vi "LVClass_ComputePhaseSet Read ComputePhaseSet.vi"(8 "error in (no error)":errorcluster, 11 "ComputePhaseSet in":refnum<class "ComputePhaseSet.lvclass">) -> (0 "error out":errorcluster, 2 "ComputePhaseSet":i32, 3 "ComputePhaseSet out":refnum<class "ComputePhaseSet.lvclass">)   [LabVIEW 2020, in "ComputePhaseSet.lvclass"]
uses:
  ComputePhaseSet.lvclass
  ComputePhaseSet.lvclass/ComputePhaseSet.ctl
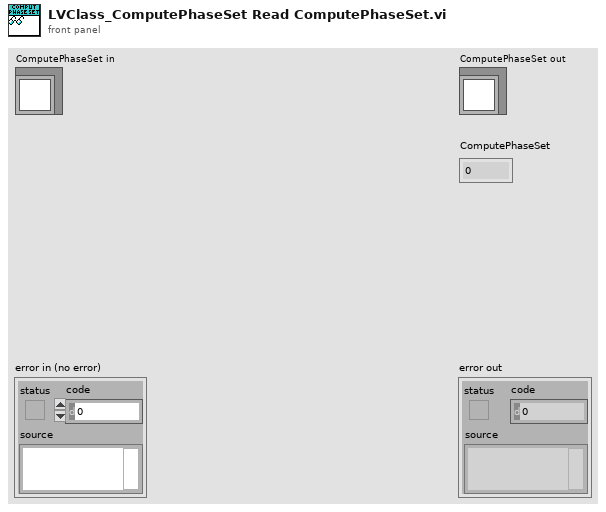
[diagram p1: front panel]
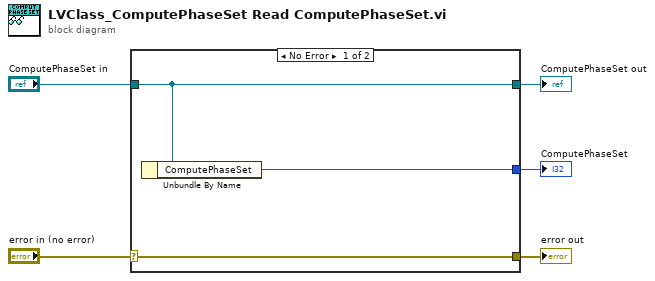
[diagram p0: block diagram]
diagram:
  n1 = case shown="No Error" "error in (no error)" {
    selector: "error in (no error)" -> [w8 w9]
    tunnel: [w8 w9] -> w4
    tunnel: [w7 w10] -> w2
    tunnel: "ComputePhaseSet in" -> [w7 w10]
    tunnel: [w6 _] -> w1
    frame No Error {
      n2 = Unbundle By Name(w7) -> ("ComputePhaseSet"=w6:i32)
    }
    frame Error {
    }
  }
  "error out" <- w4
  "ComputePhaseSet out" <- w2
  "ComputePhaseSet" <- w1
